vi "Get Vertical Step Size.vi"(8 "error in":errorcluster, 11 "eye scan in":refnum<class "niHighSpeedSerial Rectangular Eye Scan v1 Host.lvclass">) -> (0 "error out":errorcluster, 2 "vertical step size":i16, 3 "eye scan out":refnum<class "niHighSpeedSerial Rectangular Eye Scan v1 Host.lvclass">)   [LabVIEW 2014, in "niHighSpeedSerial Rectangular Eye Scan v1 Host.lvclass"]
doc: "Returns the vertical step size.\n\n<B>Input Parameters</B>\n\n<B>eye scan in</B> Takes in a reference to your session from the previous VI.\n\n<B>error in</B> describes error conditions that occur before this node runs. This input provides standard 'error in' functionality.\n\n<B>Output Parameters</B>\n\n<B>error out</B> contains error information. This output provides standard 'error out' functionality.\n\n<B>vertical step size</B> is the number of offsets to skip between each point on the vertical axis.\n\n<B>eye scan out</B> passes a reference to your session to the next VI."
uses:
  <instrlib>/niHighSpeedSerial/Eye Scan/v1/Host/Impl/Rectangular Eye Scan/niHighSpeedSerial Rectangular Eye Scan v1 Host.lvclass
  <instrlib>/niHighSpeedSerial/Eye Scan/v1/Host/Impl/Rectangular Eye Scan/niHighSpeedSerial Rectangular Eye Scan v1 Host.lvclass/niHighSpeedSerial Rectangular Eye Scan v1 Host.ctl
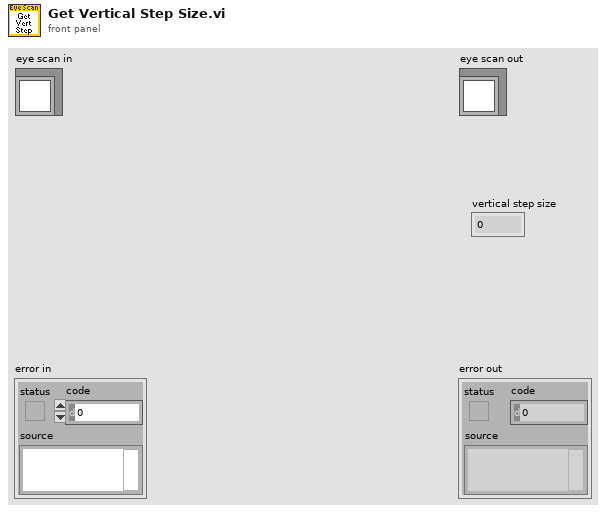
[diagram p1: front panel]
types:
  T1 = typedef "Rectangular Eye Scan v1 Host.lvclass/Private Data.ctl" = cluster{"horizontal step size":i16, "vertical step size":i16, "rectangular eye scan point iterator":refnum<class "niHighSpeedSerial Rectangular Eye Scan Point Iterator v1 Host.lvclass">}
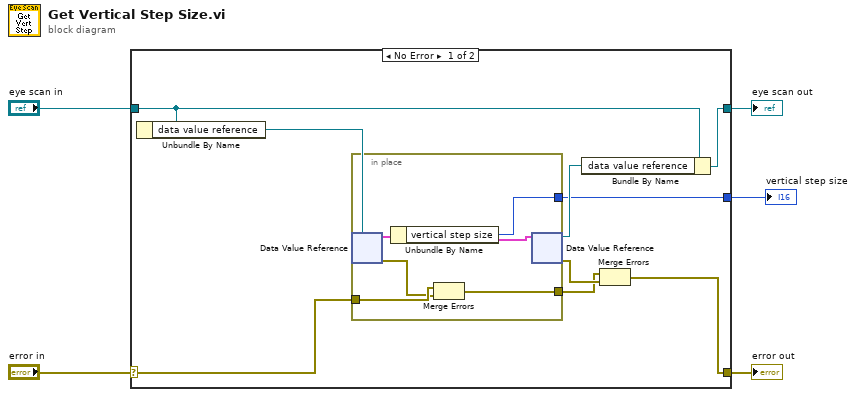
[diagram p0: block diagram]
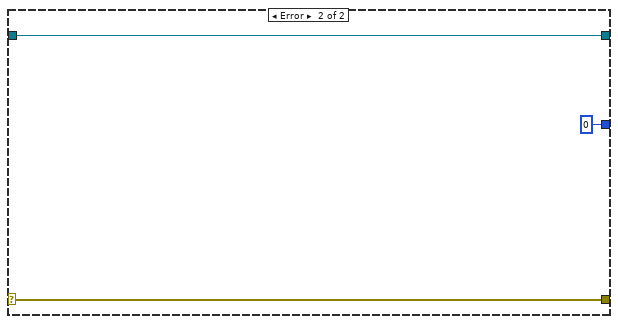
[diagram p2: hidden frame]
diagram:
  n1 = case shown="No Error" "error in" {
    selector: "error in" -> [w10 w22]
    tunnel: [w7 w22] -> w4
    tunnel: [w13 w21] -> w2
    tunnel: "eye scan in" -> [w14 w21]
    tunnel: [w6 i16 0 ("horizontal step size")] -> w1
    frame No Error {
      n2 = Unbundle By Name(w14) -> ("data value reference"=w11:refnum<data-value>)
      n3 = in-place {
        in-place-border: w10 -> [w19]
        in-place-border: [w17] -> w8
        in-place-border: [w16] -> w6
        n4 = in-place-dvr #1(w11) -> (w15:T1, w18:errorcluster)
        n5 = Unbundle By Name(w15) -> ("vertical step size"=w16:i16)
        n6 = Merge Errors(w19, w18) -> (w17:errorcluster)
        n7 = in-place-dvr #1(w15) -> (w12:refnum<data-value>, w9:errorcluster)
      }
      n8 = Bundle By Name(cluster=w14, "data value reference"=w12) -> (w13:refnum<class "niHighSpeedSerial Rectangular Eye Scan v1 Host.lvclass">)
      n9 = Merge Errors(w8, w9) -> (w7:errorcluster)
    }
    frame Error {
    }
  }
  "error out" <- w4
  "eye scan out" <- w2
  "vertical step size" <- w1
